vi "ModeMgr.Mode Setup Dialog.vi"(11 "Mode Config File":path) -> ()   [LabVIEW 2018]
uses:
  ModeMgr.Mode Settings_Config View.ctl
  ModeMgr.Mode Settings.ctl
  <vilib>/KATE/Files/File Utils.lvlib
panel:
  in  "Main Tab":enum32{"Modes", "Documentation", "Config"}(tab)
  in  "Close":bool
  in  "Modes":T1[](array[typedef])=[{"Name"="Production", "Color"=3, "Options"=[{"Option"="Can Access Station Module", "Level"=0}, {"Option"="Can Auto Repeat Sequence", "Level"=0}, {"Option"="Can Clear Errors", "Level"=0}, {"Option"="Can Clear Warnings", "Level"=0}, {"Option"="Can Edit EQ List", "Level"=0}, {"Option"="Can Edit Options", "Level"=0}, {"Option"="Can Generate Reports", "Level"=0}, {"Option"="Can Select Sequence", "Level"=0}, {"Option"="Can View Config", "Level"=0}, {"Option"="Disable Results", "Level"=0}, {"Option"="Disable Start with SN Entry", "Level"=0}, {"Option"="Display Result Data Details", "Level"=0}, {"Option"="Not Reset SN between Tests", "Level"=0}, {"Option"="Not Validate Operator", "Level"=0}, {"Option"="Not Validate SN", "Level"=0}], "Password"=""}, {"Name"="Technician", "Color"=1, "Options"=[{"Option"="Can Access Station Module", "Level"=0}, {"Option"="Can Auto Repeat Sequence", "Level"=0}, {"Option"="Can Clear Errors", "Level"=1}, {"Option"="Can Clear Warnings", "Level"=1}, {"Option"="Can Edit EQ List", "Level"=0}, {"Option"="Can Edit Options", "Level"=0}, {"Option"="Can Generate Reports", "Level"=1}, {"Option"="Can Select Sequence", "Level"=1}, {"Option"="Can View Config", "Level"=0}, {"Option"="Disable Results", "Level"=0}, {"Option"="Disable Start with SN Entry", "Level"=1}, {"Option"="Display Result Data Details", "Level"=1}, {"Option"="Not Reset SN between Tests", "Level"=1}, {"Option"="Not Validate Operator", "Level"=1}, {"Option"="Not Validate SN", "Level"=0}], "Password"=""}, {"Name"="Gage R&R", "Color"=6, "Options"=[{"Option"="Can Access Station Module", "Level"=0}, {"Option"="Can Auto Repeat Sequence", "Level"=0}, {"Option"="Can Clear Errors", "Level"=0}, {"Option"="Can Clear Warnings", "Level"=0}, {"Option"="Can Edit EQ List", "Level"=0}, {"Option"="Can Edit Options", "Level"=0}, {"Option"="Can Generate Reports", "Level"=0}, {"Option"="Can Select Sequence", "Level"=0}, {"Option"="Can View Config", "Level"=0}, {"Option"="Disable Results", "Level"=0}, {"Option"="Disable Start with SN Entry", "Level"=0}, {"Option"="Display Result Data Details", "Level"=0}, {"Option"="Not Reset SN between Tests", "Level"=0}, {"Option"="Not Validate Operator", "Level"=0}, {"Option"="Not Validate SN", "Level"=0}], "Password"=""}, {"Name"="Engineering", "Color"=4, "Options"=[{"Option"="Can Access Station Module", "Level"=1}, {"Option"="Can Auto Repeat Sequence", "Level"=1}, {"Option"="Can Clear Errors", "Level"=1}, {"Option"="Can Clear Warnings", "Level"=1}, {"Option"="Can Edit EQ List", "Level"=1}, {"Option"="Can Edit Options", "Level"=1}, {"Option"="Can Generate Reports", "Level"=1}, {"Option"="Can Select Sequence", "Level"=1}, {"Option"="Can View Config", "Level"=1}, {"Option"="Disable Results", "Level"=1}, {"Option"="Disable Start with SN Entry", "Level"=1}, {"Option"="Display Result Data Details", "Level"=1}, {"Option"="Not Reset SN between Tests", "Level"=1}, {"Option"="Not Validate Operator", "Level"=1}, {"Option"="Not Validate SN", "Level"=1}], "Password"="Pa$$word"}] {"Color" items=["Red", "Yellow", "Orange", "Green", "SkyBlue", "Blue", "Purple", "Pink", "Grey"]}
  in  "Mode List":i32(listbox)=-1
  in  "Default Mode":string="Production"
  in  "Load":bool
  in  "Save":bool
  in  "Save As":bool
  in  "Add Mode":bool
  in  "Delete Mode":bool
  in  "Dup Mode":bool
  out "Error":errorcluster
  out "Option Descriptions":cluster{"Option":string, "Desc":string}[](array[cluster])=[{"Option"="Can Access Station Module", "Desc"="Level 0 = the button and menu item to open the station control module is not available.  Level 1 (or higher) = the station module can be opened."}, {"Option"="Can Clear Errors", "Desc"="Level 0 = the button to clear errors is disabled.  Level 1 (or higher) = the button to clear errors is enabled."}, {"Option"="Can Clear Warnings", "Desc"="Level 0 = the button to clear warnings is disabled.  Level 1 (or higher) = the button to clear warnings is enabled."}, {"Option"="Can Edit EQ List", "Desc"="Level 0 = the Equipment list can not be edited.  Level 1 (or higher) = the Equipment list can be edited."}, {"Option"="Can Edit Options", "Desc"="Level 0 = the controls for options (on tab page Config - Options) is disabled.  Level 1 (or higher) = the controls for options (on tab page Config - Options) is enabled."}, {"Option"="Can Generate Reports", "Desc"="Level 0 = the controls to generate RTF or CSV reports are disabled.  Level 1 (or higher) = the controls to generate RTF or CSV reports are enabled."}, {"Option"="Can Select Sequence", "Desc"="Level 0 = the controls for selecting the test sequence is disabled.  The default sequence (configured) is the only available sequenct that can be run. Level 1 (or higher) = the sequence selector control is enabled."}, {"Option"="Can View Config", "Desc"="Level 0 = the tab page for Config is hidden.  Level 1 (or higher) = the tab page for Config is visible and can eb selected."}, {"Option"="Disable Results", "Desc"="Level 0 = test results are reported for each test 9to Factory and to Data Warehouse).  Level 1 (or higher) = no results are reported."}, {"Option"="Disable Start with SN Entry", "Desc"="Level 0 = the control to auto start test when a SN is entered is set to ON and can not be changed.  Level 1 (or higher) = the control to auto start test when a SN is entered is set to OFF and can be changed by the operator."}, {"Option"="Display Result Data Details", "Desc"="\"Level 0 =  The operator can only view the summary page.  Level 1 (or higher) = the tabs of the result section will be displayed and the operator can select to view the Summary"}, {"Option"="Not Reset SN between Tests", "Desc"="Level 0 = the SN field is cleared between tests.  Level 1 (or higher) = the SN remains the same between tests."}, {"Option"="Not Validate Operator", "Desc"="Level 0 = the operator field can not be empty.  The Start button is disabled until the operator field is populated.  Level 1 (or higher) = the operator can be empty."}, {"Option"="Not Validate SN", "Desc"="Level 0 = the SN field can not be empty.  The Start button is disabled until the SN field is populated.  Level 1 (or higher) = the SN can be empty."}]
  out "Default Config":path
  out "Options Config File":path
  out "Options":string[](array[string])=["Option", "Display Result Data Details", "Not Reset SN between Tests", "Not Validate Operator", "Not Validate SN", "Disable Results", "Can Access Station Module", "Can Edit EQ List", "Can Clear Warnings", "Can Clear Errors", "Can View Config", "Can Edit Options", "Can Select Sequence", "Can Generate Reports", "Disable Start with SN Entry"]
  # "Option                                                                                             Description"
  # "Click top right corner (X) to close"
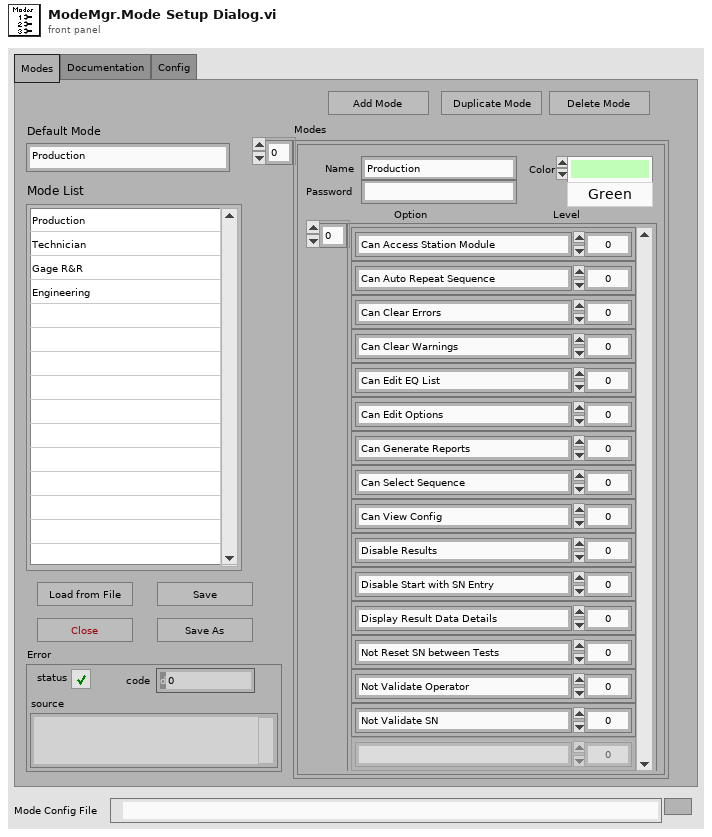
[diagram p1: front panel]
types:
  T1 = typedef "ModeMgr.Mode Settings_Config View.ctl" = cluster{"Name":string, "Color":u16, "Options":T2[], "Password":string}
  T2 = typedef "ModeMgr.Mode Settings.ctl" = cluster{"Option":string, "Level":i32}
  T3 = enum32{"invalid app kind", "Development System", "Run Time System", "Student Edition", "Embedded LabVIEW", "Evaluation", "Custom"}
  T4 = enum32{"Invalid", "Standard", "Closed", "Hidden", "Minimized", "Maximized"}
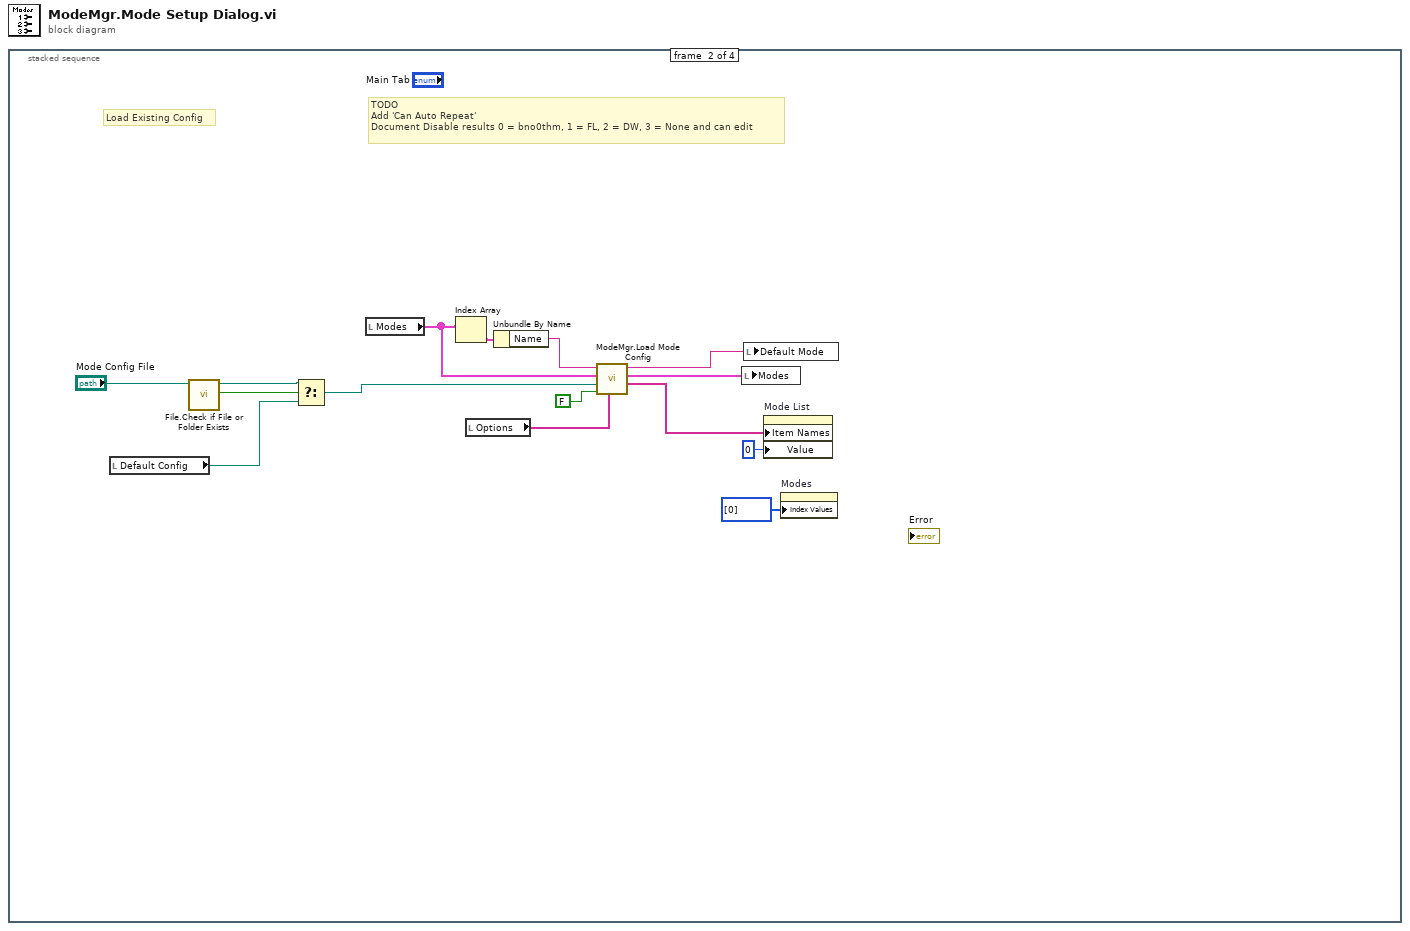
[diagram p0: block diagram]
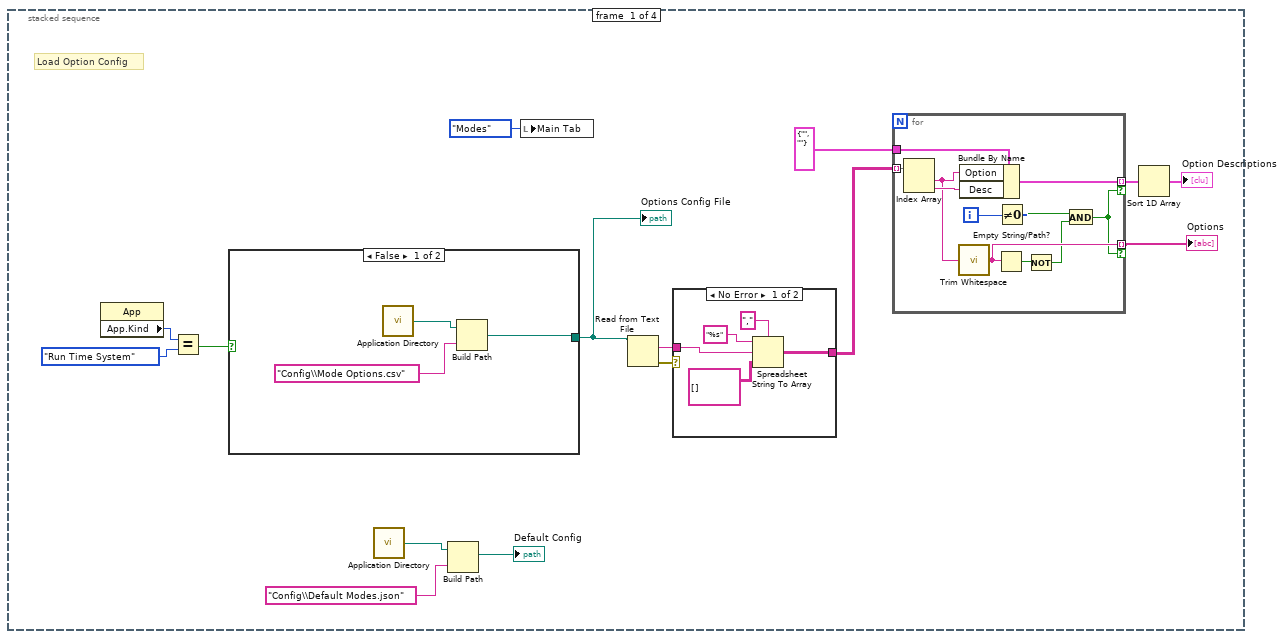
[diagram p2: hidden frame]
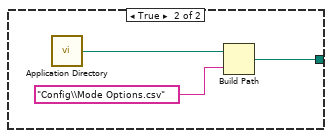
[diagram p4: hidden frame]
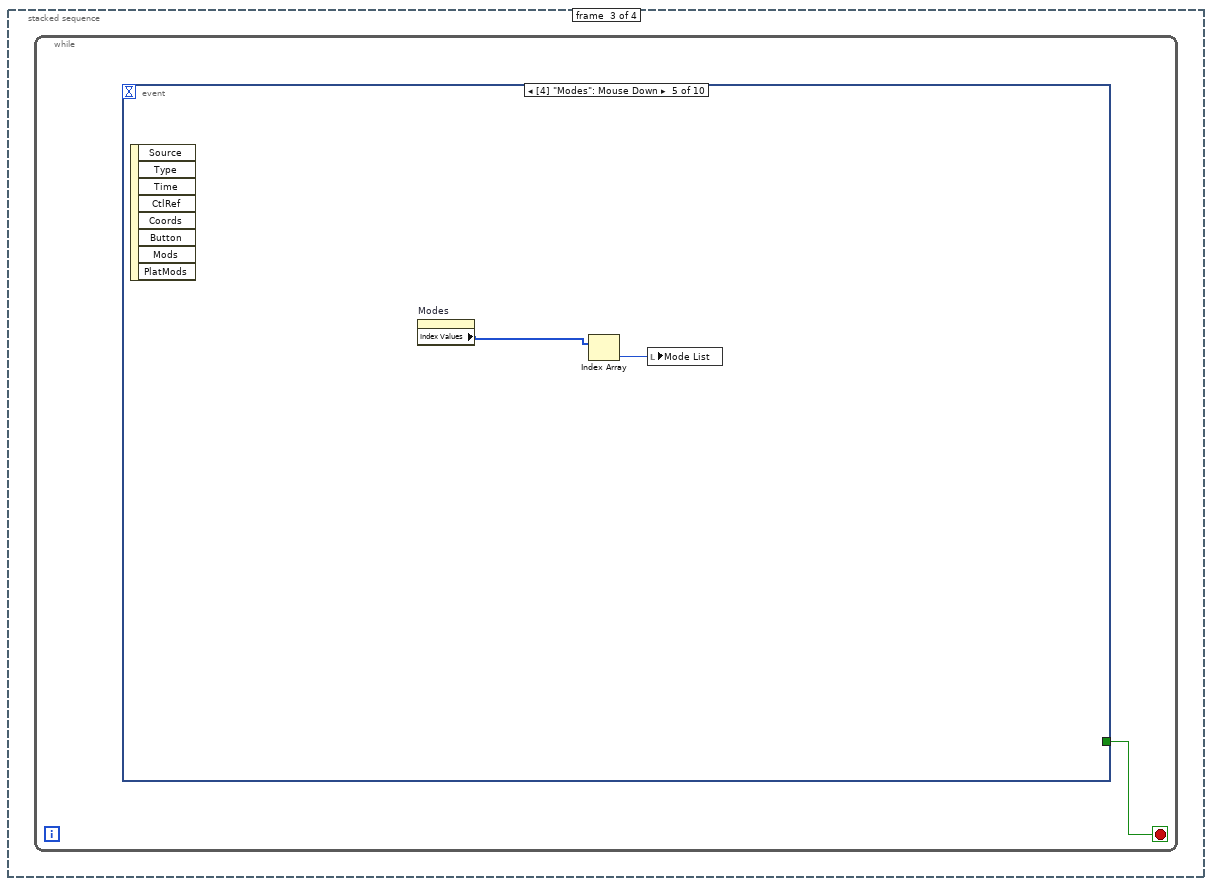
[diagram p5: hidden frame]
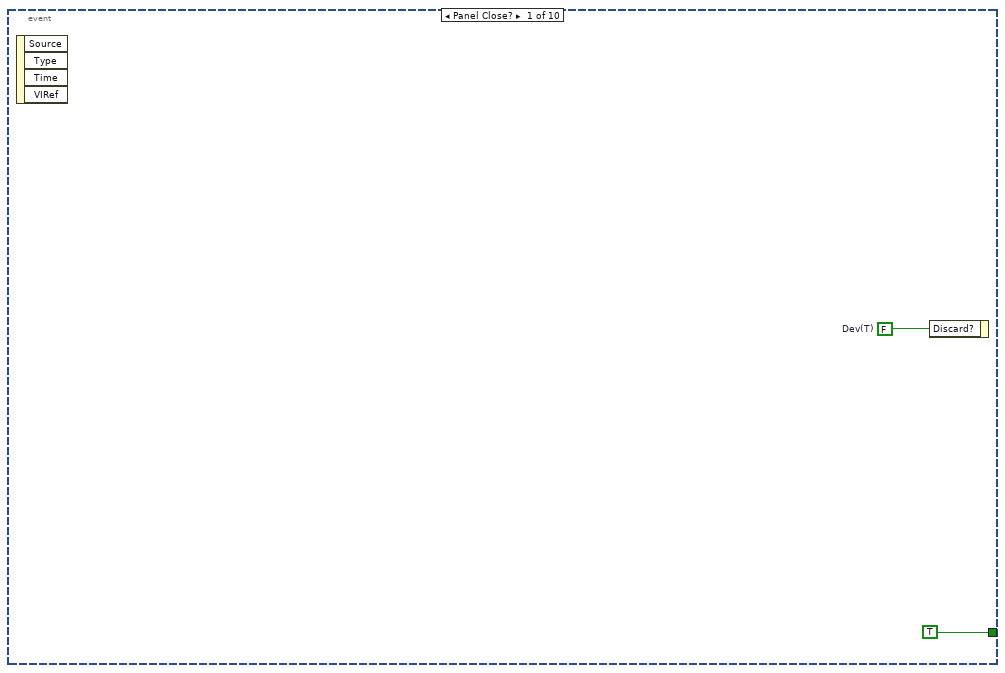
[diagram p6: hidden frame]
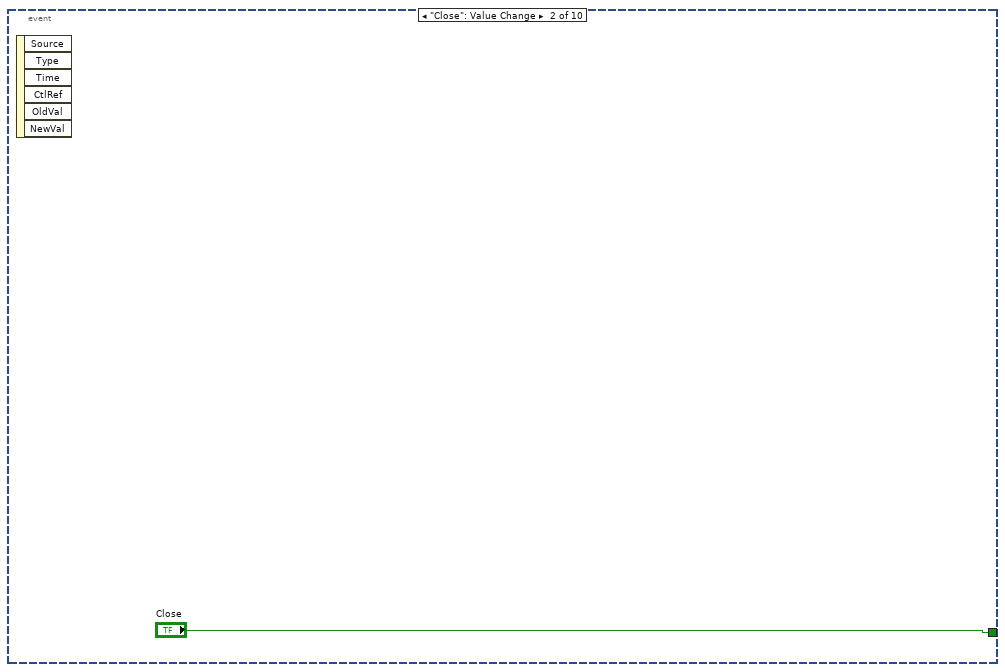
[diagram p7: hidden frame]
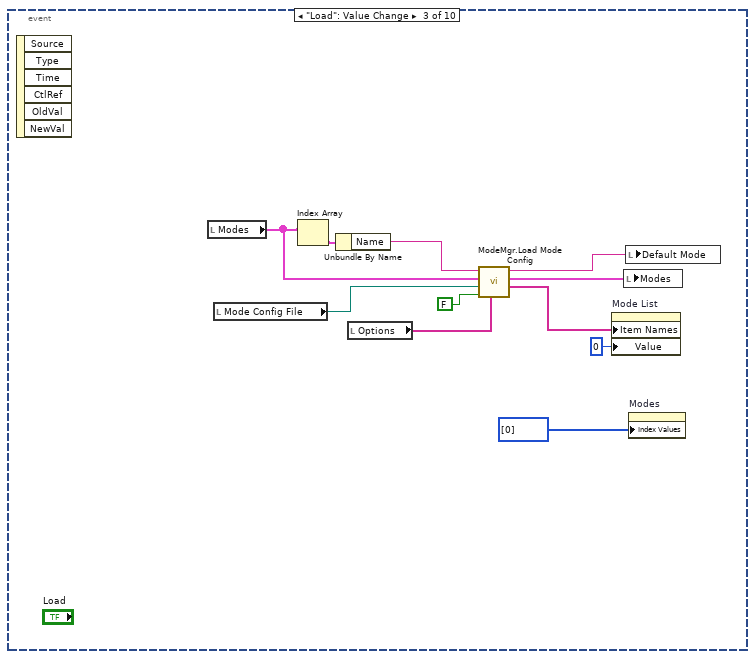
[diagram p8: hidden frame]
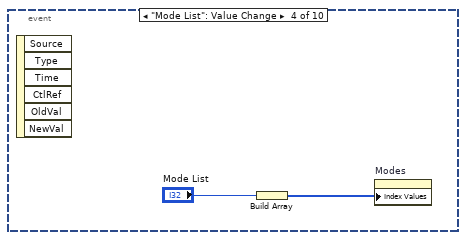
[diagram p9: hidden frame]
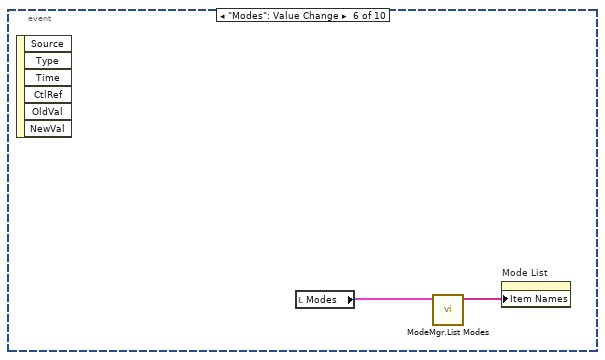
[diagram p10: hidden frame]
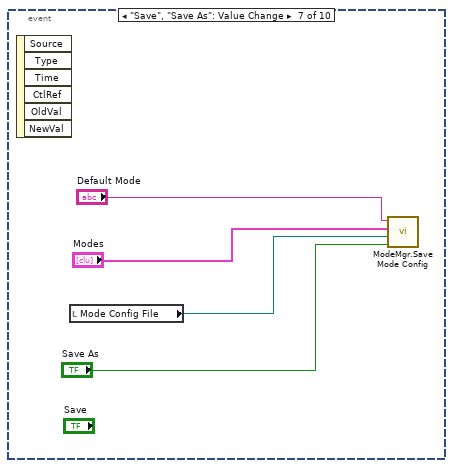
[diagram p11: hidden frame]
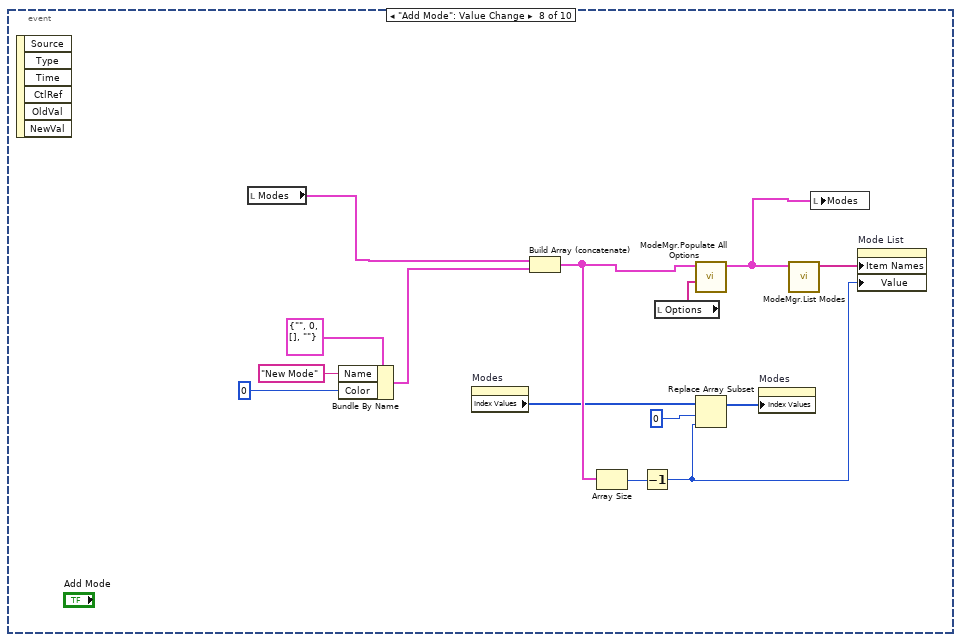
[diagram p12: hidden frame]
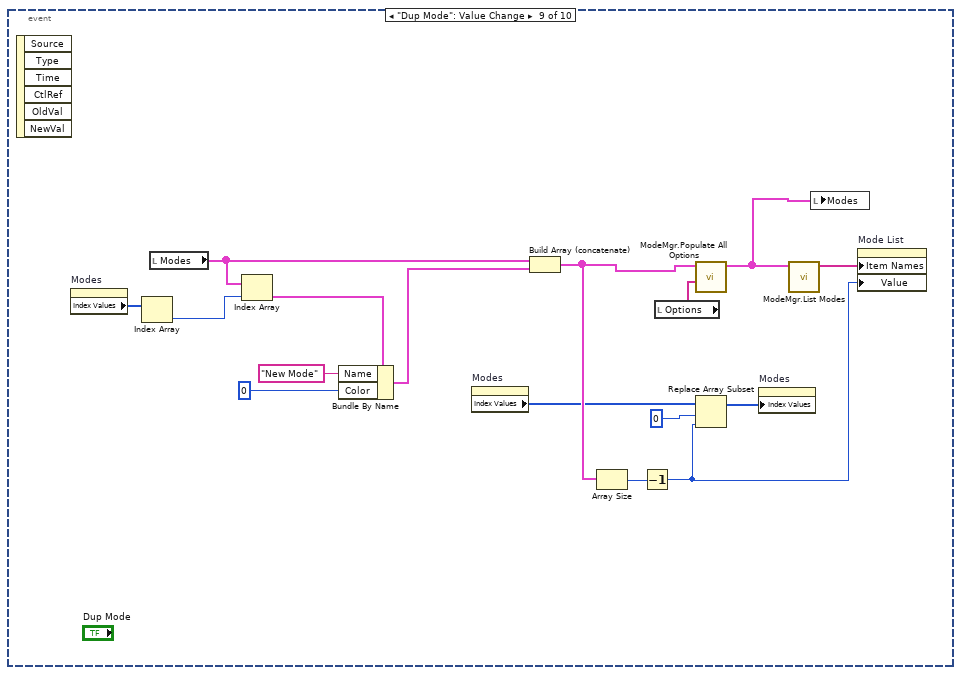
[diagram p13: hidden frame]
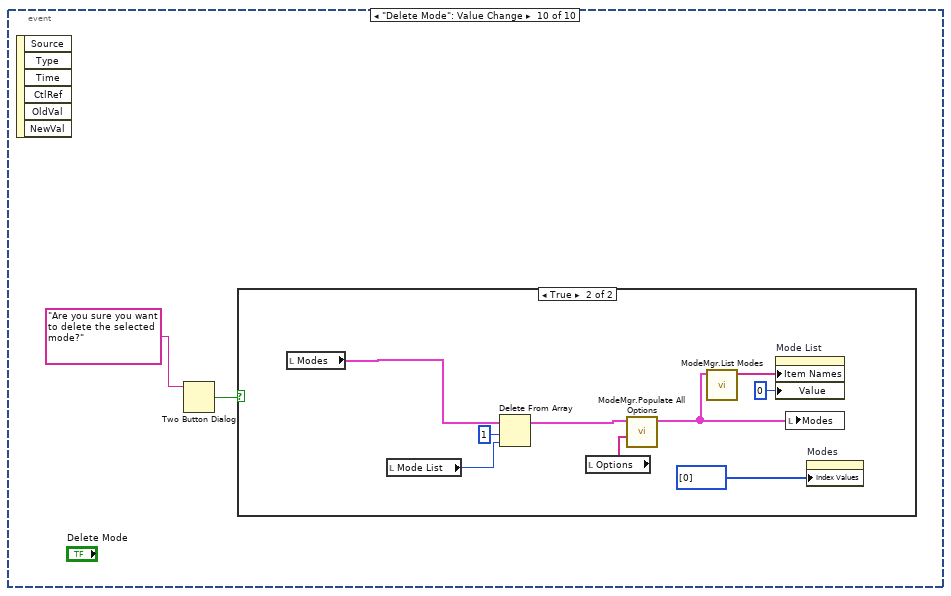
[diagram p14: hidden frame]
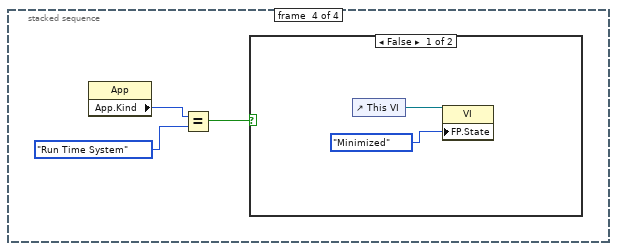
[diagram p16: hidden frame]
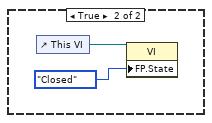
[diagram p17: hidden frame]
diagram:
  n1 = stacked-sequence {
    frame #0 {
      # "Load Option Config"
      n2 = property class="App"() -> ("App.Kind"=w15:T3)  [unwired: 2 in, 2 out]
      n3 = Equal?(x=w15, y=T3."Run Time System" ("Application:Kind")) -> (x = y?=w13:bool)
      n4 = case shown="False" w13 {
        tunnel: [w32 w35] -> w12
        frame False {
          n5 = call <vilib>:"Application Directory.vi"() -> ("Application Directory"=w33:path)
          n6 = Build Path(base path=w33, name or relative path="Config\\Mode Options.csv") -> (appended path=w32:path)
        }
        frame True {
          n7 = call <vilib>:"Application Directory.vi"() -> ("Application Directory"=w37:path)
          n8 = Build Path(base path=w37, name or relative path="Config\\Mode Options.csv") -> (appended path=w35:path)
        }
      }
      "Options Config File" <- w12
      n9 = call <vilib>:"Application Directory.vi"() -> ("Application Directory"=w3:path)
      n10 = Build Path(base path=w3, name or relative path="Config\\Default Modes.json") -> (appended path=→"Default Config":path)
      n11 = local write "Main Tab"(enum32{"Modes", "Documentation", "Config"}."Modes" ("Main Tab")) -> ()
      n12 = Read from Text File(file (use dialog)=w12) -> (text=w10:string, error out=w11:errorcluster)  [unwired: 3 in, 2 out]
      n13 = case shown="No Error" w11 {
        tunnel: w10 -> [w30 _]
        tunnel: [w27 _] -> w6
        frame No Error {
          n14 = Spreadsheet String To Array(delimiter (Tab)=",", format string="%s", spreadsheet string=w30, array type (2D Dbl)=string[][] []) -> (array=w27:string[][])
        }
        frame Error {
        }
      }
      n15 = for {
        tunnel: w6 -> [w25] mode=indexing
        tunnel: cluster{"Option":string, "Desc":string} {"Option"="", "Desc"=""} ("Cluster") -> [w26]
        tunnel: [w24] -> w8 mode=indexing if=w16
        tunnel: [w19] -> w4 mode=indexing if=w16
        i -> [w22]
        n16 = Index Array(array=w25) -> (element #1=w21:string, element #2=w23:string)  [unwired: 2 in]
        n17 = call <vilib>:"Trim Whitespace.vi"("string"=w21) -> ("trimmed string"=w19:string)  [unwired: 1 in]
        n18 = Bundle By Name(cluster=w26, "Option"=w21, "Desc"=w23) -> (w24:cluster{"Option":string, "Desc":string})
        n19 = Empty String/Path?(string/path=w19) -> (empty?=w20:bool)
        n20 = Not Equal To 0?(x=w22) -> (x != 0?=w18:bool)
        n21 = Not(x=w20) -> (.not. x?=w17:bool)
        n22 = And(x=w18, y=w17) -> (x .and. y?=w16:bool)
      }
      "Options" <- w4
      n23 = Sort 1D Array(array=w8) -> (sorted array=→"Option Descriptions":cluster{"Option":string, "Desc":string}[])
    }
    frame #1 {
      # "TODO\nAdd 'Can Auto Repeat'\nDocument Disable results 0 = bno0thm, 1 = FL, 2 = DW, 3 = None and can edit"
      # "Load Existing Config"
      n24 = local read "Default Config"() -> (w39:path)
      n25 = call <vilib>:"File.Check if File or Folder Exists.vi"("Path"="Mode Config File") -> ("Exists"=w40:bool, "Dup Path"=w41:path)  [unwired: 6 in, 3 out]
      n26 = Select(t=w41, s=w40, f=w39) -> (s? t:f=w38:path)
      n27 = local read "Modes"() -> (w51:T1[])
      n28 = Index Array(array=w51) -> (element=w50:T1)  [unwired: 1 in]
      n29 = local read "Options"() -> (w48:string[])
      n30 = Unbundle By Name(w50) -> ("Name"=w49:string)
      n31 = call "ModeMgr.Load Mode Config.vi"("Options"=w48, "Use DIalog"=FALSE, "Path"=w38, "Modes"=w51, "Default Mode"=w49) -> ("Names"=w44:string[], "Modes Out"=w47:T1[], "Default Mode Out"=w46:string)  [unwired: 3 in, 1 out]
      n32 = local write "Modes"(w47) -> ()
      n33 = local write "Default Mode"(w46) -> ()
      n34 = property on="Mode List" class="LstBox (strict)"("Item Names"=w44, "Value"=0 ("Modes")) -> ()  [unwired: 2 in, 2 out]
      n35 = property on="Modes" class="Arr (strict)"("Index Values"=u32[] [0]) -> ()  [unwired: 2 in, 2 out]
    }
    frame #2 {
      n36 = while {
        stop <- w53 stop-if-true
        n37 = event shown="[4] \"Modes\": Mouse Down" {
          selector: _ -> [_ _ _ _ _ _ _ _ _ _]
          dyn-events: _ -> [_ _ _ _ _ _ _ _ _ _]
          timeout: _ -> [_ _ _ _ _ _ _ _ _ _]
          tunnel: [TRUE "Close" _ _ _ _ _ _ _ _] -> w53
          event Panel Close? {
            w54 = FALSE  # Dev(T)
            n38 = event-data() -> ()  [unwired: 1 in, 4 out]
            n39 = event-data("Discard?"=w54) -> ()  [unwired: 1 in, 1 out]
          }
          event "Close": Value Change {
            n40 = event-data() -> ()  [unwired: 1 in, 6 out]
          }
          event "Load": Value Change {
            n41 = event-data() -> ()  [unwired: 1 in, 6 out]
            n42 = local read "Modes"() -> (w66:T1[])
            n43 = local read "Mode Config File"() -> (w67:path)
            n44 = Index Array(array=w66) -> (element=w65:T1)  [unwired: 1 in]
            n45 = Unbundle By Name(w65) -> ("Name"=w64:string)
            n46 = local read "Options"() -> (w63:string[])
            n47 = call "ModeMgr.Load Mode Config.vi"("Options"=w63, "Use DIalog"=FALSE, "Path"=w67, "Modes"=w66, "Default Mode"=w64) -> ("Names"=w60:string[], "Modes Out"=w62:T1[], "Default Mode Out"=w61:string)  [unwired: 3 in, 1 out]
            n48 = property on="Mode List" class="LstBox (strict)"("Item Names"=w60, "Value"=0 ("Modes")) -> ()  [unwired: 2 in, 2 out]
            n49 = local write "Modes"(w62) -> ()
            n50 = local write "Default Mode"(w61) -> ()
            n51 = property on="Modes" class="Arr (strict)"("Index Values"=u32[] [0]) -> ()  [unwired: 2 in, 2 out]
          }
          event "Mode List": Value Change {
            n52 = event-data() -> ()  [unwired: 1 in, 6 out]
            n53 = Build Array("Mode List") -> (w68:i32[])
            n54 = property on="Modes" class="Arr (strict)"("Index Values"=w68) -> ()  [unwired: 2 in, 2 out]
          }
          event "Modes": Mouse Down {
            n55 = event-data() -> ()  [unwired: 1 in, 8 out]
            n56 = property on="Modes" class="Arr (strict)"() -> ("Index Values"=w70:u32[])  [unwired: 2 in, 2 out]
            n57 = Index Array(array=w70) -> (element=w71:u32)  [unwired: 1 in]
            n58 = local write "Mode List"(w71) -> ()
          }
          event "Modes": Value Change {
            n59 = event-data() -> ()  [unwired: 1 in, 6 out]
            n60 = local read "Modes"() -> (w73:T1[])
            n61 = call "ModeMgr.List Modes.vi"("Modes"=w73) -> ("Names"=w72:string[])  [unwired: 10 in]
            n62 = property on="Mode List" class="LstBox (strict)"("Item Names"=w72) -> ()  [unwired: 2 in, 2 out]
          }
          event "Save", "Save As": Value Change {
            n63 = event-data() -> ()  [unwired: 1 in, 6 out]
            n64 = local read "Mode Config File"() -> (w74:path)
            n65 = call "ModeMgr.Save Mode Config.vi"("Use DIalog"="Save As", "Path"=w74, "Modes"="Modes", "Default Mode"="Default Mode") -> ()  [unwired: 8 in]
          }
          event "Add Mode": Value Change {
            n66 = event-data() -> ()  [unwired: 1 in, 6 out]
            n67 = local read "Modes"() -> (w81:T1[])
            n68 = Bundle By Name(cluster=T1 {"Name"="", "Color"=0, "Options"=[], "Password"=""} ("Config"), "Name"="New Mode", "Color"=u16 0) -> (w89:T1)
            n69 = property on="Modes" class="Arr (strict)"() -> ("Index Values"=w79:u32[])  [unwired: 2 in, 2 out]
            n70 = Build Array (concatenate)(w81, w89) -> (w80:T1[])
            n71 = Array Size(array=w80) -> (size(s)=w84:i32)
            n72 = Decrement(x=w84) -> (x-1=w83:i32)
            n73 = local read "Options"() -> (w86:string[])
            n74 = call "ModeMgr.Populate All Options.vi"("Options"=w86, "Modes"=w80) -> ("Modes Out"=w85:T1[])  [unwired: 9 in]
            n75 = Replace Array Subset(array=w79, new element=w83, index=0) -> (w78:u32[])
            n76 = property on="Modes" class="Arr (strict)"("Index Values"=w78) -> ()  [unwired: 2 in, 2 out]
            n77 = call "ModeMgr.List Modes.vi"("Modes"=w85) -> ("Names"=w90:string[])  [unwired: 10 in]
            n78 = local write "Modes"(w85) -> ()
            n79 = property on="Mode List" class="LstBox (strict)"("Item Names"=w90, "Value"=w83) -> ()  [unwired: 2 in, 2 out]
          }
          event "Dup Mode": Value Change {
            n80 = event-data() -> ()  [unwired: 1 in, 6 out]
            n81 = property on="Modes" class="Arr (strict)"() -> ("Index Values"=w93:u32[])  [unwired: 2 in, 2 out]
            n82 = Index Array(array=w93) -> (element=w92:u32)  [unwired: 1 in]
            n83 = local read "Modes"() -> (w95:T1[])
            n84 = Index Array(array=w95, index=w92) -> (element=w94:T1)
            n85 = Bundle By Name(cluster=w94, "Name"="New Mode", "Color"=u16 0) -> (w105:T1)
            n86 = property on="Modes" class="Arr (strict)"() -> ("Index Values"=w97:u32[])  [unwired: 2 in, 2 out]
            n87 = Build Array (concatenate)(w95, w105) -> (w98:T1[])
            n88 = Array Size(array=w98) -> (size(s)=w100:i32)
            n89 = Decrement(x=w100) -> (x-1=w99:i32)
            n90 = local read "Options"() -> (w102:string[])
            n91 = call "ModeMgr.Populate All Options.vi"("Options"=w102, "Modes"=w98) -> ("Modes Out"=w101:T1[])  [unwired: 9 in]
            n92 = Replace Array Subset(array=w97, new element=w99, index=0) -> (w96:u32[])
            n93 = property on="Modes" class="Arr (strict)"("Index Values"=w96) -> ()  [unwired: 2 in, 2 out]
            n94 = call "ModeMgr.List Modes.vi"("Modes"=w101) -> ("Names"=w106:string[])  [unwired: 10 in]
            n95 = local write "Modes"(w101) -> ()
            n96 = property on="Mode List" class="LstBox (strict)"("Item Names"=w106, "Value"=w99) -> ()  [unwired: 2 in, 2 out]
          }
          event "Delete Mode": Value Change {
            n97 = event-data() -> ()  [unwired: 1 in, 6 out]
            n98 = Two Button Dialog(message="Are you sure you want to delete the selected mode?") -> (T button?=w108:bool)  [unwired: 2 in]
            n99 = case shown="True" w108 {
              frame False {
              }
              frame True {
                n100 = local read "Modes"() -> (w112:T1[])
                n101 = local read "Mode List"() -> (w117:i32)
                n102 = Delete From Array(array=w112, length=1, index=w117) -> (array with subset deleted=w111:T1[])  [unwired: 1 out]
                n103 = local read "Options"() -> (w116:string[])
                n104 = call "ModeMgr.Populate All Options.vi"("Options"=w116, "Modes"=w111) -> ("Modes Out"=w113:T1[])  [unwired: 9 in]
                n105 = call "ModeMgr.List Modes.vi"("Modes"=w113) -> ("Names"=w115:string[])  [unwired: 10 in]
                n106 = property on="Mode List" class="LstBox (strict)"("Item Names"=w115, "Value"=0 ("Modes")) -> ()  [unwired: 2 in, 2 out]
                n107 = local write "Modes"(w113) -> ()
                n108 = property on="Modes" class="Arr (strict)"("Index Values"=u32[] [0]) -> ()  [unwired: 2 in, 2 out]
              }
            }
          }
        }
      }
    }
    frame #3 {
      n109 = property class="App"() -> ("App.Kind"=w121:T3)  [unwired: 2 in, 2 out]
      n110 = Equal?(x=w121, y=T3."Run Time System" ("Application:Kind")) -> (x = y?=w119:bool)
      n111 = case shown="False" w119 {
        frame False {
          n112 = control-ref of="This VI"() -> (w123:refnum<vi>)
          n113 = property class="VI"(reference=w123, "FP.State"=T4."Minimized" ("Front Panel Window:State")) -> ()  [unwired: 1 in, 2 out]
        }
        frame True {
          n114 = control-ref of="This VI"() -> (w125:refnum<vi>)
          n115 = property class="VI"(reference=w125, "FP.State"=T4."Closed" ("Front Panel Window:State")) -> ()  [unwired: 1 in, 2 out]
        }
      }
    }
  }
